vi "Load_And_Intitiate_Velocity.vi"() -> ()   [LabVIEW 2018]
panel:
  out "Serial Out":refnum<visa-resource-name>
  out "Error Out":errorcluster
  in  "Error In":errorcluster
  in  "Serial In":refnum<visa-resource-name>
  in  "Relative?":bool
  in  "Position":i64
  in  "Node":i32
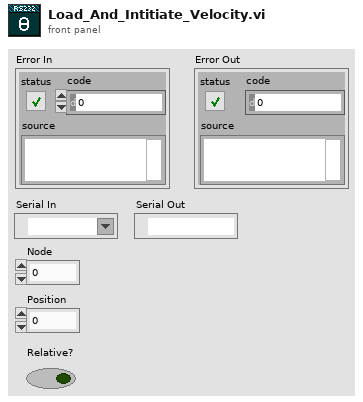
[diagram p1: front panel]
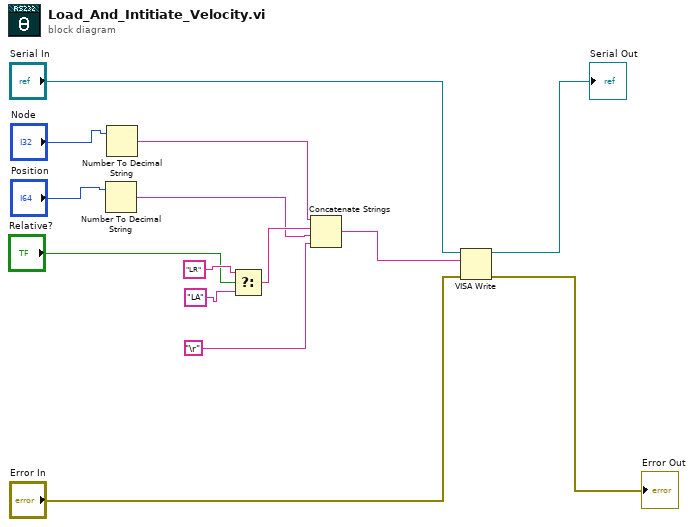
[diagram p0: block diagram]
diagram:
  n1 = Number To Decimal String(number="Position") -> (decimal integer string=w2:string)  [unwired: 1 in]
  n2 = Number To Decimal String(number="Node") -> (decimal integer string=w4:string)  [unwired: 1 in]
  n3 = Select(t="LR", s="Relative?", f="LA") -> (s? t:f=w3:string)
  n4 = Concatenate Strings(w4, w3, w2, "\r") -> (w1:string)
  n5 = VISA Write(VISA resource name="Serial In", write buffer=w1, error in (no error)="Error In") -> (VISA resource name out=→"Serial Out":refnum<visa-resource-name>, error out=→"Error Out":errorcluster)  [unwired: 1 out]
